vi "testError.vi"() -> ()   [LabVIEW 2019, in "AssertionTest.lvlib" / "AssertNotEquals.lvlib"]
uses:
  AssertNotEquals.lvlib
  0715dcc1-2d30-44c5-a3a2-e455403ccc4a.vi
  <vilib>/Utility/error.llb/Error Cluster From Error Code.vi
  Constraint/IsEqual/Create.vi
  <vilib>/ErrorRing/Error Ring.xnode
  Constraint/IsEqual/IsEqual.lvclass
  a742ccf2-dc70-4a69-b295-5438a718dbcf.vi
panel:
  out "error out":errorcluster
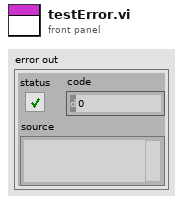
[diagram p1: front panel]
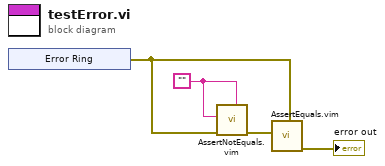
[diagram p0: block diagram]
diagram:
  w1 = ""
  n1 = xnode "Error Ring"() -> ("error out"=w2:errorcluster)
  n2 = call "AssertNotEquals.vim"("Expected"=w1, "error in (no error)"=w2, "Actual"=w1) -> ("error out"=w4:errorcluster)  [unwired: 8 in]
  n3 = call "AssertEquals.vim"("Expected"=w2, "Actual"=w4) -> ("error out"=→"error out":errorcluster)  [unwired: 9 in]
